vi "Delete DIOs RT FIFO.vi"(8 "error in":errorcluster, 11 "DIOs RT FIFO":refnum<k33>) -> (0 "error out":errorcluster)   [LabVIEW 2021, in "RT Main.lvlib"]
uses:
  RT Main.lvlib
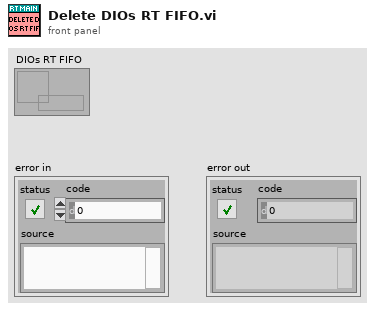
[diagram p1: front panel]
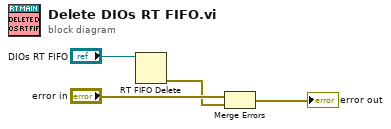
[diagram p0: block diagram]
diagram:
  n1 = RT FIFO Delete(0:"DIOs RT FIFO") -> (11:w2:errorcluster)  [unwired: 2 in]
  n2 = Merge Errors("error in", w2) -> (→"error out":errorcluster)
